vi "Serve Schedules.vi"(11 "LabVIEW Web Service Request":refnum<class "Web Request.lvclass">) -> ()   [LabVIEW 2013]
uses:
  <vilib>/wsapi/Web Request.lvclass
  <vilib>/xml/Close Reference(Node).vi
  <vilib>/xml/NI_XML.lvlib
  <resource>/objmgr/DOMUserDefRef.rc
panel:
  out "XML":string
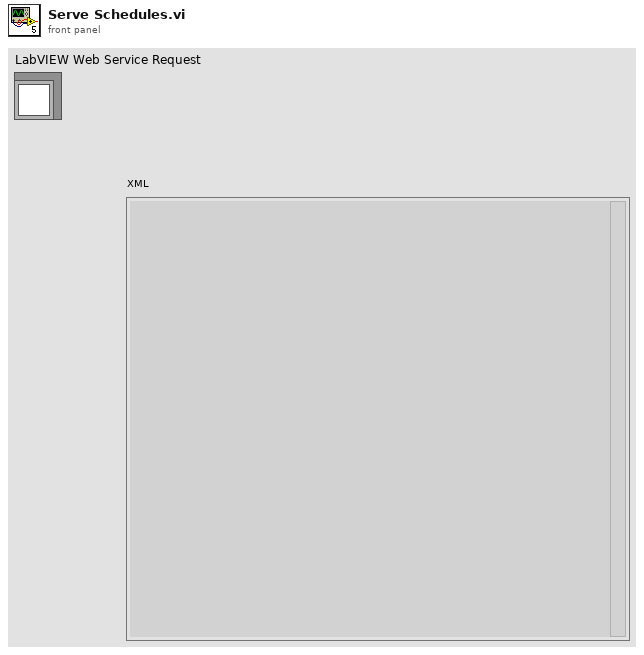
[diagram p1: front panel]
types:
  T1 = typedef "Schedule Data.ctl" = cluster{"Practice Matches":string[][], "Ranking Matches":string[][], "Table Names":string[], "Ranking Match Times":string[][], "Practice Match Times":string[][]}
  T2 = cluster{"Practice Match Times[0]":string, "Practice Match Times[1]":string, "Practice Match Times[2]":string, "Practice Match Times[3]":string, "Practice Match Times[4]":string, "Practice Match Times[5]":string, "Practice Match Times[6]":string, "Practice Match Times[7]":string, "Practice Match Times[8]":string}
  T3 = cluster{"Ranking Match Times[0]":string, "Ranking Match Times[1]":string, "Ranking Match Times[2]":string, "Ranking Match Times[3]":string, "Ranking Match Times[4]":string, "Ranking Match Times[5]":string, "Ranking Match Times[6]":string, "Ranking Match Times[7]":string, "Ranking Match Times[8]":string}
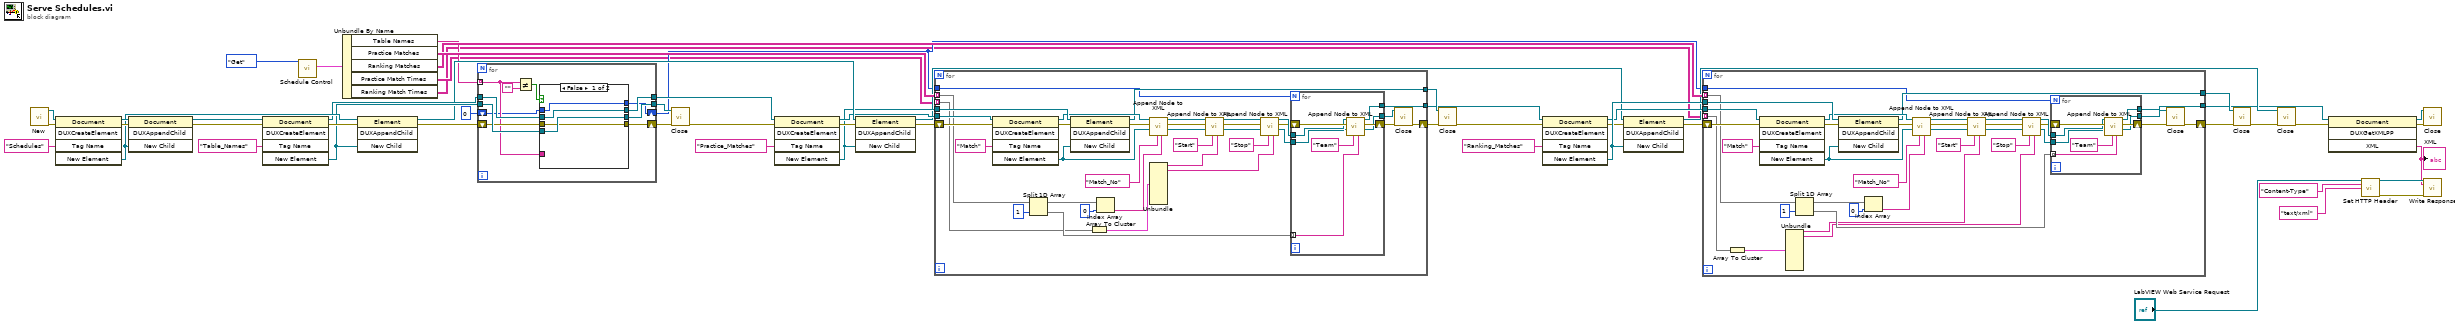
[diagram p0: block diagram]
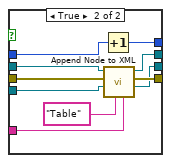
[diagram p2: hidden frame]
diagram:
  n1 = call <vilib>:"New.vi"() -> ("error out"=w54:errorcluster, "DOM document out"=w55:refnum<k20>)  [unwired: 8 in]
  n2 = invoke class="Document" method="DUXCreateElement"(reference=w55, error in=w54, "Tag Name"="Schedules") -> (reference out=w52:refnum<k20>, error out=w51:errorcluster, "New Element"=w46:refnum<k20>)  [unwired: 2 in, 2 out]
  n3 = invoke class="Document" method="DUXAppendChild"(reference=w52, error in=w51, "New Child"=w46) -> (reference out=w50:refnum<k20>, error out=w49:errorcluster)  [unwired: 1 in, 2 out]
  n4 = invoke class="Document" method="DUXCreateElement"(reference=w50, error in=w49, "Tag Name"="Table_Names") -> (reference out=w45:refnum<k20>, error out=w47:errorcluster, "New Element"=w43:refnum<k20>)  [unwired: 2 in, 2 out]
  n5 = call "Schedule Control.vi"("Mode"=enum16{"Get", "Set"}."Get") -> ("Schedule Data Out"=w42:T1)  [unwired: 10 in]
  n6 = Unbundle By Name(w42) -> ("Table Names"=w11:string[], "Practice Matches"=w34:string[][], "Ranking Matches"=w21:string[][], "Practice Match Times"=w2:string[][], "Ranking Match Times"=w1:string[][])
  n7 = invoke class="Element" method="DUXAppendChild"(reference=w46, error in=w47, "New Child"=w43) -> (reference out=w36:refnum<k20>, error out=w44:errorcluster)  [unwired: 1 in, 2 out]
  n8 = for {
    tunnel: w45 -> [w67]
    shift-right: [w63] -> w41
    shift-left: w44 -> [w65]
    tunnel: w43 -> [w66]
    tunnel: w11 -> [w61] mode=indexing
    tunnel: [w64] -> w39
    tunnel: [w62] -> w40
    shift-right: [w57] -> w9
    shift-left: 0 -> [w58]
    n9 = Not Equal?(x=w61, y="") -> (x != y?=w59:bool)
    n10 = case shown="False" w59 {
      tunnel: w67 -> [w71 w81]
      tunnel: w66 -> [w70 w80]
      tunnel: w65 -> [w69 w79]
      tunnel: w61 -> [_ w77]
      tunnel: [w71 w76] -> w64
      tunnel: [w69 w75] -> w63
      tunnel: [w70 w74] -> w62
      tunnel: w58 -> [w68 w73]
      tunnel: [w68 w72] -> w57
      frame False {
      }
      frame True {
        n11 = Increment(x=w73) -> (x+1=w72:i32)
        n12 = call "Append Node to XML.vi"("Data"=w77, "Tag Name"="Table", "SuperElement In"=w80, "error in"=w79, "DOM document in"=w81) -> ("SuperElement Out"=w74:refnum<k20>, "error out"=w75:errorcluster, "DOM document out"=w76:refnum<k20>)  [unwired: 4 in]
      }
    }
  }
  n13 = call-poly <vilib>:"Close.vi"("error in (no error)"=w41, "node"=w40) -> ("error out"=w38:errorcluster)  [unwired: 7 in]
  n14 = invoke class="Document" method="DUXCreateElement"(reference=w39, error in=w38, "Tag Name"="Practice_Matches") -> (reference out=w33:refnum<k20>, error out=w35:errorcluster, "New Element"=w31:refnum<k20>)  [unwired: 2 in, 2 out]
  n15 = invoke class="Element" method="DUXAppendChild"(reference=w36, error in=w35, "New Child"=w31) -> (reference out=w22:refnum<k20>, error out=w32:errorcluster)  [unwired: 1 in, 2 out]
  n16 = for {
    tunnel: w34 -> [w101] mode=indexing
    tunnel: w33 -> [w116]
    shift-right: [w106] -> w12
    shift-left: w32 -> [w115]
    tunnel: w31 -> [w113]
    tunnel: [w105] -> w30
    tunnel: [w104] -> w19
    tunnel: w9 -> [w103]
    tunnel: w2 -> [w85] mode=indexing
    n17 = invoke class="Document" method="DUXCreateElement"(reference=w116, error in=w115, "Tag Name"="Match") -> (reference out=w110:refnum<k20>, error out=w112:errorcluster, "New Element"=w111:refnum<k20>)  [unwired: 2 in, 2 out]
    n18 = Split 1D Array(array=w101, index=1) -> (first subarray=w99:string[], second subarray=w100:string[])
    n19 = invoke class="Element" method="DUXAppendChild"(reference=w113, error in=w112, "New Child"=w111) -> (reference out=w105:refnum<k20>, error out=w109:errorcluster)  [unwired: 1 in, 2 out]
    n20 = Array To Cluster(array=w85) -> (cluster=w84:T2)
    n21 = Index Array(array=w99, index=0) -> (element=w97:string)
    n22 = call "Append Node to XML.vi"("Data"=w97, "Tag Name"="Match_No", "SuperElement In"=w111, "error in"=w109, "DOM document in"=w110) -> ("SuperElement Out"=w91:refnum<k20>, "error out"=w92:errorcluster, "DOM document out"=w93:refnum<k20>)  [unwired: 4 in]
    n23 = Unbundle(w84) -> ("Practice Match Times[0]"=w83:string, "Practice Match Times[1]"=w82:string)  [unwired: 7 out]
    n24 = call "Append Node to XML.vi"("Data"=w83, "Tag Name"="Start", "SuperElement In"=w91, "error in"=w92, "DOM document in"=w93) -> ("SuperElement Out"=w96:refnum<k20>, "error out"=w94:errorcluster, "DOM document out"=w95:refnum<k20>)  [unwired: 4 in]
    n25 = call "Append Node to XML.vi"("Data"=w82, "Tag Name"="Stop", "SuperElement In"=w96, "error in"=w94, "DOM document in"=w95) -> ("SuperElement Out"=w89:refnum<k20>, "error out"=w88:errorcluster, "DOM document out"=w90:refnum<k20>)  [unwired: 4 in]
    n26 = for {
      N: w103 -> [_]
      shift-right: [w120] -> w108
      shift-left: w88 -> [w125]
      tunnel: w100 -> [w118] mode=indexing
      tunnel: w90 -> [w124]
      tunnel: w89 -> [w123]
      tunnel: [w121] -> w104
      tunnel: [w119] -> w107
      n27 = call "Append Node to XML.vi"("Data"=w118, "Tag Name"="Team", "SuperElement In"=w123, "error in"=w125, "DOM document in"=w124) -> ("SuperElement Out"=w119:refnum<k20>, "error out"=w120:errorcluster, "DOM document out"=w121:refnum<k20>)  [unwired: 4 in]
    }
    n28 = call-poly <vilib>:"Close.vi"("error in (no error)"=w108, "node"=w107) -> ("error out"=w106:errorcluster)  [unwired: 7 in]
  }
  n29 = call-poly <vilib>:"Close.vi"("error in (no error)"=w12, "node"=w30) -> ("error out"=w20:errorcluster)  [unwired: 7 in]
  n30 = invoke class="Document" method="DUXCreateElement"(reference=w19, error in=w20, "Tag Name"="Ranking_Matches") -> (reference out=w25:refnum<k20>, error out=w24:errorcluster, "New Element"=w27:refnum<k20>)  [unwired: 2 in, 2 out]
  n31 = invoke class="Element" method="DUXAppendChild"(reference=w22, error in=w24, "New Child"=w27) -> (reference out=w18:refnum<k20>, error out=w26:errorcluster)  [unwired: 1 in, 2 out]
  n32 = for {
    tunnel: w21 -> [w145] mode=indexing
    tunnel: w25 -> [w160]
    shift-right: [w150] -> w28
    shift-left: w26 -> [w159]
    tunnel: w27 -> [w157]
    tunnel: [w149] -> w29
    tunnel: [w148] -> w16
    tunnel: w9 -> [w147]
    tunnel: w1 -> [w129] mode=indexing
    n33 = Array To Cluster(array=w129) -> (cluster=w128:T3)
    n34 = invoke class="Document" method="DUXCreateElement"(reference=w160, error in=w159, "Tag Name"="Match") -> (reference out=w154:refnum<k20>, error out=w156:errorcluster, "New Element"=w155:refnum<k20>)  [unwired: 2 in, 2 out]
    n35 = Unbundle(w128) -> ("Ranking Match Times[0]"=w127:string, "Ranking Match Times[1]"=w126:string)  [unwired: 7 out]
    n36 = Split 1D Array(array=w145, index=1) -> (first subarray=w142:string[], second subarray=w144:string[])
    n37 = invoke class="Element" method="DUXAppendChild"(reference=w157, error in=w156, "New Child"=w155) -> (reference out=w149:refnum<k20>, error out=w153:errorcluster)  [unwired: 1 in, 2 out]
    n38 = Index Array(array=w142, index=0) -> (element=w141:string)
    n39 = call "Append Node to XML.vi"("Data"=w141, "Tag Name"="Match_No", "SuperElement In"=w155, "error in"=w153, "DOM document in"=w154) -> ("SuperElement Out"=w133:refnum<k20>, "error out"=w134:errorcluster, "DOM document out"=w137:refnum<k20>)  [unwired: 4 in]
    n40 = call "Append Node to XML.vi"("Data"=w127, "Tag Name"="Start", "SuperElement In"=w133, "error in"=w134, "DOM document in"=w137) -> ("SuperElement Out"=w139:refnum<k20>, "error out"=w138:errorcluster, "DOM document out"=w140:refnum<k20>)  [unwired: 4 in]
    n41 = call "Append Node to XML.vi"("Data"=w126, "Tag Name"="Stop", "SuperElement In"=w139, "error in"=w138, "DOM document in"=w140) -> ("SuperElement Out"=w132:refnum<k20>, "error out"=w135:errorcluster, "DOM document out"=w136:refnum<k20>)  [unwired: 4 in]
    n42 = for {
      N: w147 -> [_]
      shift-right: [w163] -> w152
      shift-left: w135 -> [w169]
      tunnel: w144 -> [w165] mode=indexing
      tunnel: w136 -> [w168]
      tunnel: w132 -> [w167]
      tunnel: [w164] -> w148
      tunnel: [w162] -> w151
      n43 = call "Append Node to XML.vi"("Data"=w165, "Tag Name"="Team", "SuperElement In"=w167, "error in"=w169, "DOM document in"=w168) -> ("SuperElement Out"=w162:refnum<k20>, "error out"=w163:errorcluster, "DOM document out"=w164:refnum<k20>)  [unwired: 4 in]
    }
    n44 = call-poly <vilib>:"Close.vi"("error in (no error)"=w152, "node"=w151) -> ("error out"=w150:errorcluster)  [unwired: 7 in]
  }
  n45 = call-poly <vilib>:"Close.vi"("error in (no error)"=w28, "node"=w29) -> ("error out"=w17:errorcluster)  [unwired: 7 in]
  n46 = call-poly <vilib>:"Close.vi"("error in (no error)"=w17, "node"=w18) -> ("error out"=w15:errorcluster)  [unwired: 7 in]
  n47 = invoke class="Document" method="DUXGetXMLPP"(reference=w16, error in=w15) -> (reference out=w14:refnum<k20>, error out=w13:errorcluster, "XML"=w6:string)  [unwired: 2 in, 1 out]
  "XML" <- w6
  n48 = call <vilib>:"Set HTTP Header.vi"("LabVIEW Web Service Request"="LabVIEW Web Service Request", "header"="Content-Type", "header value"="text/xml") -> ("LabVIEW Web Service Request out"=w8:refnum<class "Web Request.lvclass">, "error out"=w7:errorcluster)  [unwired: 11 in]
  n49 = call-poly <vilib>:"Close.vi"("error in (no error)"=w13, "node"=w14) -> ()  [unwired: 7 in, 1 out]
  n50 = call <vilib>:"Write Response.vi"("LabVIEW Web Service Request"=w8, "response string"=w6, "error in (no error)"=w7) -> ()  [unwired: 11 in, 2 out]
